vi "Front panel Controls.vi"(8 "error in":errorcluster, 10 "Front Panel Control (W)":T1, 11 "Write/Read":enum16{"Write", "Read"}(ring)=enum."Read") -> (0 "error out":errorcluster, 2 "Front Panel Control (R)":T1)   [LabVIEW 2022 SP3]
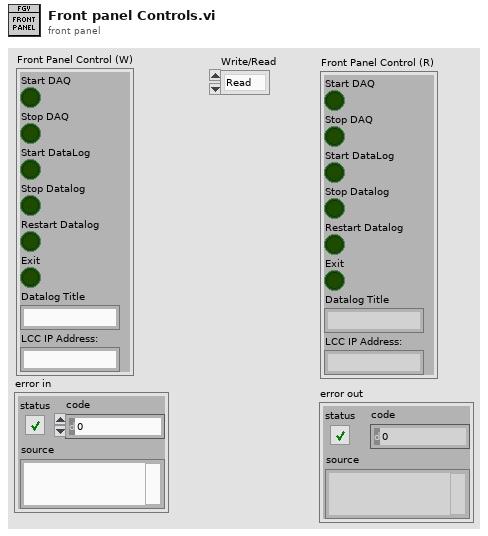
[diagram p1: front panel]
types:
  T1 = cluster{"Start DAQ":bool, "Stop DAQ":bool, "Start DataLog":bool, "Stop Datalog":bool, "Restart Datalog ":bool, "Exit":bool, "Datalog Title":string, "LCC IP Address:":string}
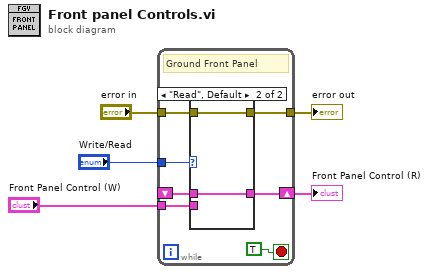
[diagram p0: block diagram]
diagram:
  n1 = while {
    tunnel: "Front Panel Control (W)" -> [w12]
    shift-right: [w11] -> w4
    shift-left: _ -> [w10]
    tunnel: "Write/Read" -> [w9]
    tunnel: "error in" -> [w7]
    tunnel: [w6] -> w1
    stop <- TRUE stop-if-true
    # "Ground Front Panel"
    n2 = case shown="\"Read\", Default" w9 {
      tunnel: w12 -> [w14 _]
      tunnel: [w14 w16] -> w11
      tunnel: w10 -> [_ w16]
      tunnel: w7 -> [w13 w15]
      tunnel: [w13 w15] -> w6
      frame "Write" {
      }
      frame "Read", Default {
      }
    }
  }
  "Front Panel Control (R)" <- w4
  "error out" <- w1
